vi "Untitled 12.vi"() -> ()   [LabVIEW 2023]
uses:
  #typedef1.ctl
panel:
  in  "Action":T1
  out "Time Elapsed[ms]":u32
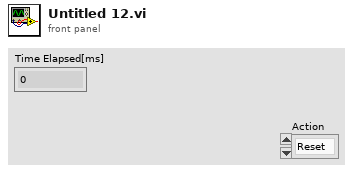
[diagram p1: front panel]
types:
  T1 = typedef "#typedef1.ctl" = enum16{"Reset", "Pause", "Run"}
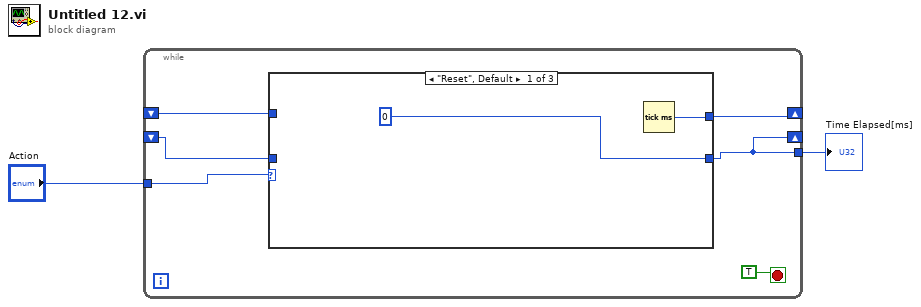
[diagram p0: block diagram]
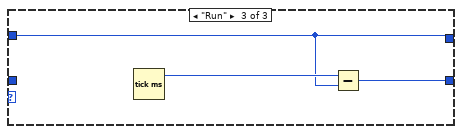
[diagram p3: hidden frame]
diagram:
  n1 = while {
    shift-right: [w7] -> _
    shift-left: _ -> [w6]
    tunnel: "Action" -> [w8]
    tunnel: [w4] -> w1
    shift-right: [w4] -> _
    shift-left: _ -> [w3]
    stop <- TRUE stop-if-true
    n2 = case shown="\"Reset\", Default" w8 {
      tunnel: [w9 w12 w14] -> w7
      tunnel: w6 -> [_ w12 w14]
      tunnel: [0 w11 w13] -> w4
      tunnel: w3 -> [_ w11 _]
      frame "Reset", Default {
        n3 = Tick Count (ms)() -> (millisecond timer value=w9:u32)
      }
      frame "Pause" {
      }
      frame "Run" {
        n4 = Tick Count (ms)() -> (millisecond timer value=w15:u32)
        n5 = Subtract(x=w15, y=w14) -> (x-y=w13:u32)
      }
    }
  }
  "Time Elapsed[ms]" <- w1
